vi "Controller Open Ethercat Variables.vi"(8 "error in (no error)":errorcluster, 11 "FOFB Configuration":T3={"FOFB Parameters"={"Network"={"FOFB Controller IP"="", "LNLS Control Network IP"="", "LNLS Control Network Power Supplies TCP Port"=0, "LNLS Control Network FOFB Configuration TCP Port"=0, "Data Server TCP Port"=0, "Monitoring Data TCP Port"=0, "Configuration GUI TCP Port"=0, "TCP Listening Timeout"=0}, "Fast Acquisition"={"Acquisition Period"=0, "Data Buffer Size"=0, "Monitoring Period"=0}, "Response Matrix Measurement"={"Step Amplitude"=0.0, "Time Between Steps"=0, "Step Duration"=0, "Number of Averages"=0}, "Correction Algorithm"={"Correction Period"=0, "Reference Orbit Path"=path "", "Response Matrix Path"=path "", "Correction Matrix Path"=path "", "Horizontal Correction Factor"=0.0, "Vertical Correction Factor"=0.0, "Beam Current FOFB Threshold"=0.0, "Decouple H-V"=FALSE, "Use Additional BPM LPF"=FALSE, "BPM LPF Cutoff"=0.0}, "Acquisition Network"=[], "Actuation Network"=[]}, "Number of Acquisition Chassis"=0, "Number of Actuation Chassis"=0, "Number of BPM Readings"=0, "BPM Reading Names"=[], "Selected BPM Readings"=[0, 1, 2, 3, 4, 5, 6, 7, 8, 9, 10, 11, 12, 13, 14, 15, 16, 17, 18, 19, 20, 21, 22, 23, 24, 25, 26, 27, 28, 29, 30, 31, 32, 33, 34, 35, 36, 37, 38, 39, 40, 41, 42, 43, 44, 45, 46, 47, 48, 49], "Number of Correctors"=0, "Corrector Names"=[], "Selected Correctors"=[0, 1, 2, 3, 4, 5, 6, 7, 8, 9, 10, 11, 12, 13, 14, 15, 16, 17, 18, 19, 20, 21, 22, 23, 24, 25, 26, 27, 28, 29, 30, 31, 32, 33, 34, 35, 36, 37, 38, 39, 40, 41, 42, 43, 44, 45, 46, 47, 48, 49], "Reference Orbit"=[], "Response Matrix"=[], "Correction Matrix"=[], "Acquisition Chassis Names"=[], "Actuation Chassis Names"=[], "Acquisition Variables"=[], "Actuation Variables"=[], "PS Matrix Mapping"=[], "Inverse PS Matrix Mapping"=[], "Response Matrix Beam Energy (MeV)"=0.0, "PID Parameters"=[], "BPM Planes"=[], "Corrector Planes"=[], "RMM Step Factor"=[]}) -> (0 "error out":errorcluster, 2 "PS Variables":T1, 3 "BPM Variables":T2)   [LabVIEW 2011, in "Controller VIs.lvlib"]
doc: "Open references for all Acquisition and Actuation variables which are used to exchange data between the FOFB Controller and the Acquisition/Actuation chassis via the EtherCAT networks."
uses:
  Controller VIs.lvlib
  Types Definitions/Type FOFB Configuration.ctl
  Types Definitions/Type FOFB Parameters.ctl
  Types Definitions/Type Network Configuration.ctl
  Types Definitions/Type FA Configuration.ctl
  Types Definitions/Type Response Matrix Measurement Configuration.ctl
  Types Definitions/Type Correction Algorithm Configuration.ctl
  Types Definitions/Type Acquisition Network Configuration.ctl
  Types Definitions/Type Actuation Network Configuration.ctl
  Types Definitions/Type PID Parameters.ctl
  Types Definitions/Type BPM Variables.ctl
  Types Definitions/Type PS Variables.ctl
  Type Definitions.lvlib
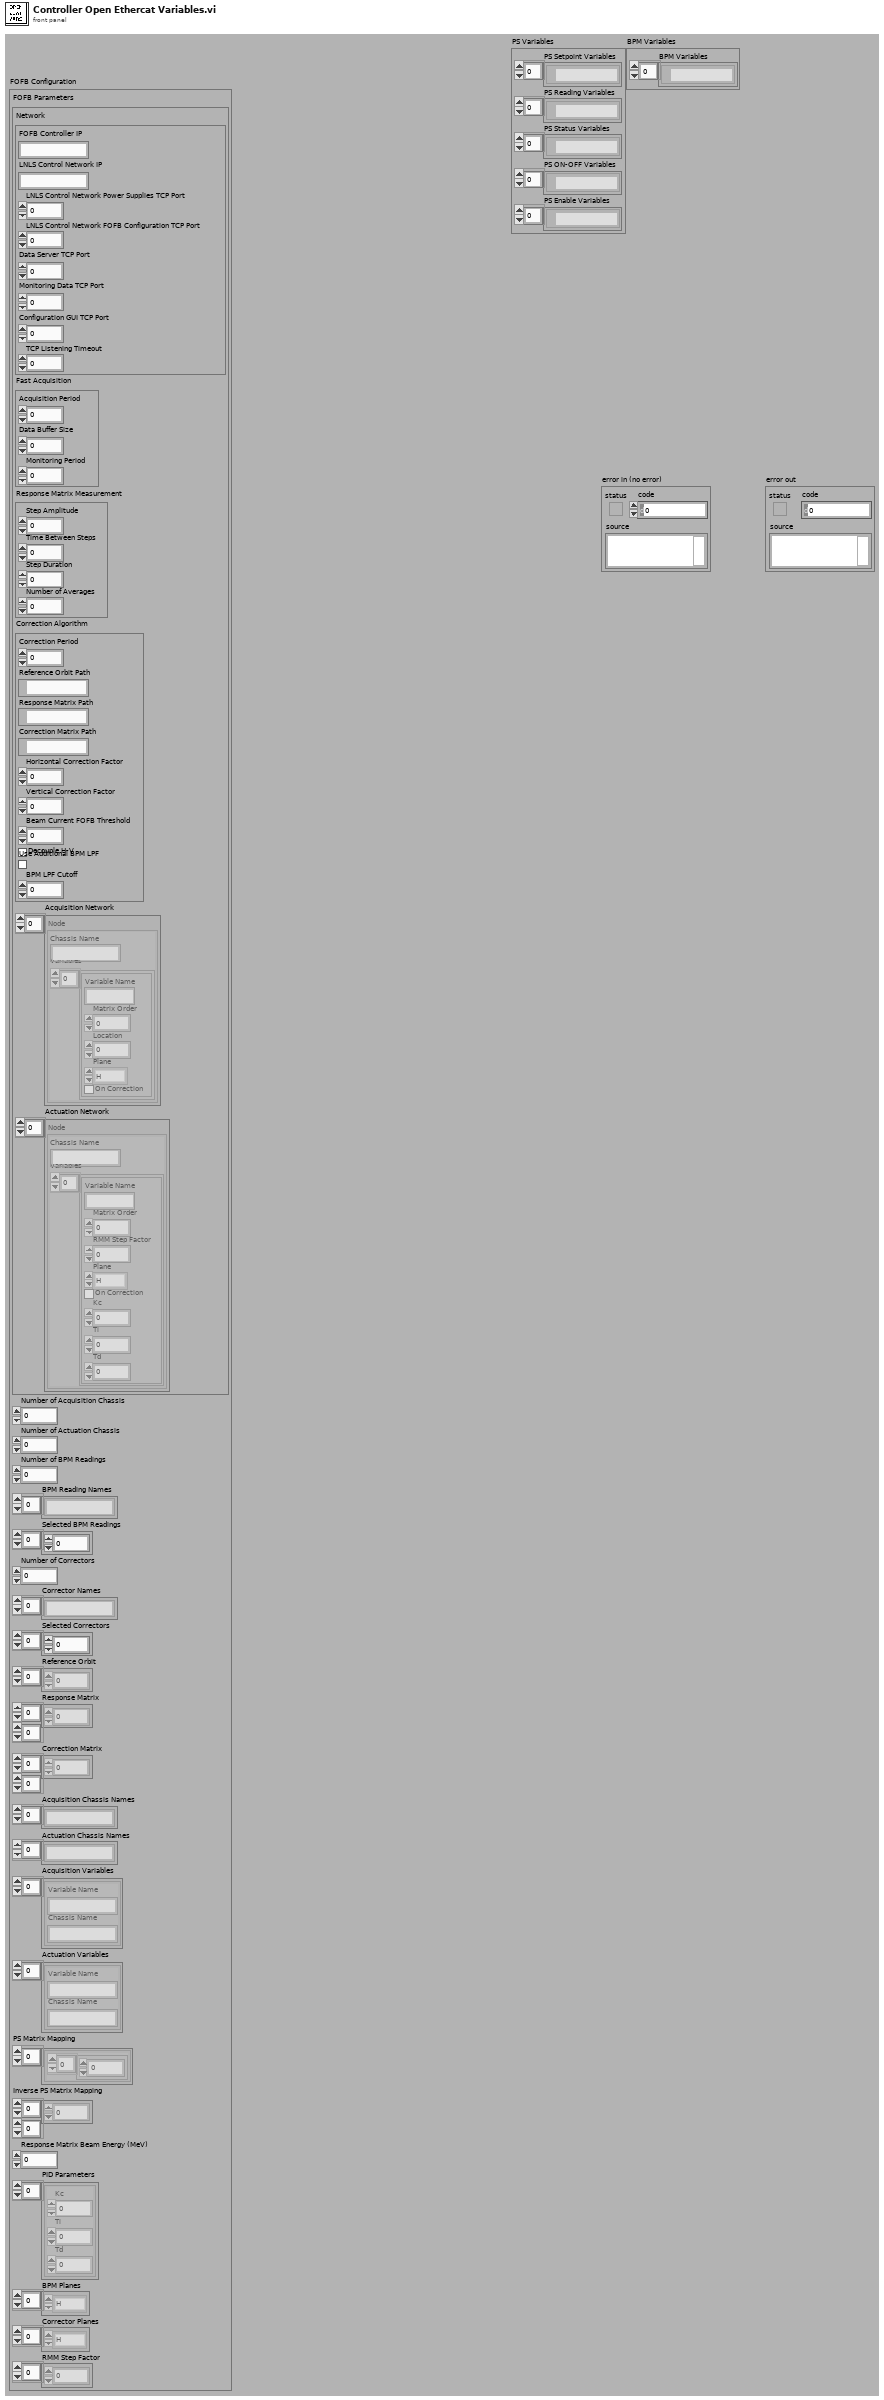
[diagram p1: front panel]
types:
  T1 = typedef "Type Definitions.lvlib/Type PS Variables.ctl" = cluster{"PS Setpoint Variables":refnum<k21>[], "PS Reading Variables":refnum<k21>[], "PS Status Variables":refnum<k21>[], "PS ON-OFF Variables":refnum<k21>[], "PS Enable Variables":refnum<k21>[]}
  T2 = typedef "Type Definitions.lvlib/Type BPM Variables.ctl" = cluster{"BPM Variables":refnum<k21>[]}
  T3 = typedef "Type Definitions.lvlib/Type FOFB Configuration.ctl" = cluster{"FOFB Parameters":T4, "Number of Acquisition Chassis":i32, "Number of Actuation Chassis":i32, "Number of BPM Readings":i32, "BPM Reading Names":string[], "Selected BPM Readings":u32[], "Number of Correctors":i32, "Corrector Names":string[], "Selected Correctors":u32[], "Reference Orbit":dbl[], "Response Matrix":dbl[][], "Correction Matrix":dbl[][], "Acquisition Chassis Names":string[], "Actuation Chassis Names":string[], "Acquisition Variables":cluster{"Variable Name":string, "Chassis Name":string}[], "Actuation Variables":cluster{"Variable Name":string, "Chassis Name":string}[], "PS Matrix Mapping":cluster{u32[]}[], "Inverse PS Matrix Mapping":u32[][], "Response Matrix Beam Energy (MeV)":dbl, "PID Parameters":T11[], "BPM Planes":enum8{"H", "V"}[], "Corrector Planes":enum8{"H", "V"}[], "RMM Step Factor":dbl[]}
  T4 = typedef "Type Definitions.lvlib/Type FOFB Parameters.ctl" = cluster{"Network":T5, "Fast Acquisition":T6, "Response Matrix Measurement":T7, "Correction Algorithm":T8, "Acquisition Network":T9, "Actuation Network":T10}
  T5 = typedef "Type Definitions.lvlib/Type Network Configuration.ctl" = cluster{"FOFB Controller IP":string, "LNLS Control Network IP":string, "LNLS Control Network Power Supplies TCP Port":u16, "LNLS Control Network FOFB Configuration TCP Port":u16, "Data Server TCP Port":u16, "Monitoring Data TCP Port":u16, "Configuration GUI TCP Port":u16, "TCP Listening Timeout":i32}
  T6 = typedef "Type Definitions.lvlib/Type FA Configuration.ctl" = cluster{"Acquisition Period":u32, "Data Buffer Size":u32, "Monitoring Period":u32}
  T7 = typedef "Type Definitions.lvlib/Type Response Matrix Measurement Configuration.ctl" = cluster{"Step Amplitude":dbl, "Time Between Steps":u32, "Step Duration":u32, "Number of Averages":u32}
  T8 = typedef "Type Definitions.lvlib/Type Correction Algorithm Configuration.ctl" = cluster{"Correction Period":u32, "Reference Orbit Path":path, "Response Matrix Path":path, "Correction Matrix Path":path, "Horizontal Correction Factor":dbl, "Vertical Correction Factor":dbl, "Beam Current FOFB Threshold":dbl, "Decouple H-V":bool, "Use Additional BPM LPF":bool, "BPM LPF Cutoff":dbl}
  T9 = typedef "Type Definitions.lvlib/Type Acquisition Network Configuration.ctl" = cluster{"Chassis Name":string, "Variables":cluster{"Variable Name":string, "Matrix Order":u32, "Location":dbl, "Plane":enum8{"H", "V"}, "On Correction":bool}[]}[]
  T10 = typedef "Type Definitions.lvlib/Type Actuation Network Configuration.ctl" = cluster{"Chassis Name":string, "Variables":cluster{"Variable Name":string, "Matrix Order":u32, "RMM Step Factor":dbl, "Plane":enum8{"H", "V"}, "On Correction":bool, "Kc":dbl, "Ti":dbl, "Td":dbl}[]}[]
  T11 = typedef "Type Definitions.lvlib/Type PID Parameters.ctl" = cluster{"Kc":fxp<+/-,16,8>, "Ti":fxp<+/-,16,8>, "Td":fxp<+/-,16,8>}
  T12 = cluster{"Variable Name":string, "Chassis Name":string}[]
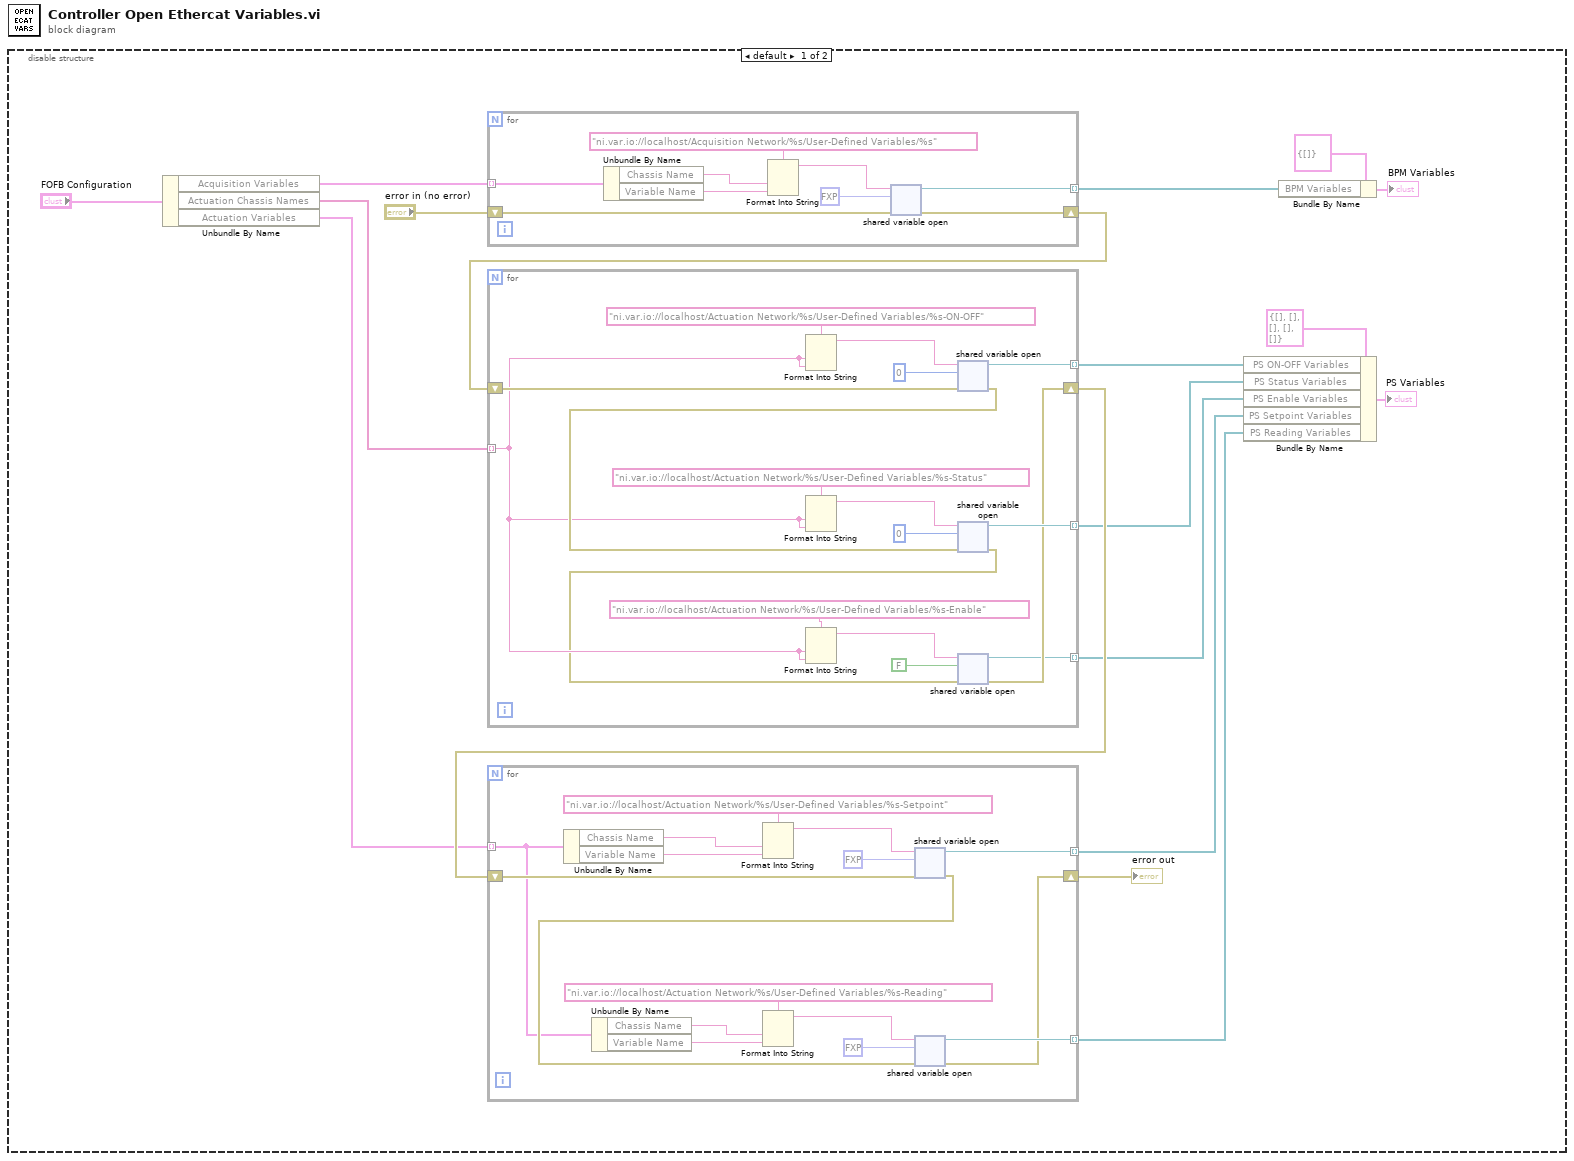
[diagram p0: block diagram]
diagram:
  n1 = disable-structure shown="default" {
    frame condition #0 {
      n2 = Unbundle By Name("FOFB Configuration") -> ("Acquisition Variables"=w8:T12, "Actuation Chassis Names"=w7:string[], "Actuation Variables"=w6:T12)
      n3 = for {
        tunnel: w8 -> [w54] mode=indexing
        shift-right: [w59] -> w13
        shift-left: "error in (no error)" -> [w58]
        tunnel: [w57] -> w17 mode=indexing
        n4 = Unbundle By Name(w54) -> ("Chassis Name"=w53:string, "Variable Name"=w52:string)
        n5 = Format Into String(format string="ni.var.io://localhost/Acquisition Network/%s/User-Defined Variables/%s", w53, w52) -> (resulting string=w56:string)  [unwired: 2 in, 1 out]
        n6 = shared-variable-open(w56, w58, fxp<+/-,20,5> 0.0 ("BPM Data")) -> (w57:refnum<k21>, w59:errorcluster)  [unwired: 1 in]
      }
      n7 = for {
        shift-right: [w20] -> w12
        shift-left: w13 -> [w28]
        tunnel: w7 -> [w22] mode=indexing
        tunnel: [w27] -> w11 mode=indexing
        tunnel: [w26] -> w10 mode=indexing
        tunnel: [w19] -> w3 mode=indexing
        n8 = Format Into String(format string="ni.var.io://localhost/Actuation Network/%s/User-Defined Variables/%s-ON-OFF", w22, w22) -> (resulting string=w35:string)  [unwired: 2 in, 1 out]
        n9 = Format Into String(format string="ni.var.io://localhost/Actuation Network/%s/User-Defined Variables/%s-Status", w22, w22) -> (resulting string=w32:string)  [unwired: 2 in, 1 out]
        n10 = Format Into String(format string="ni.var.io://localhost/Actuation Network/%s/User-Defined Variables/%s-Enable", w22, w22) -> (resulting string=w24:string)  [unwired: 2 in, 1 out]
        n11 = shared-variable-open(w35, w28, u8 0) -> (w27:refnum<k21>, w31:errorcluster)  [unwired: 1 in]
        n12 = shared-variable-open(w32, w31, u8 0) -> (w26:refnum<k21>, w21:errorcluster)  [unwired: 1 in]
        n13 = shared-variable-open(w24, w21, FALSE) -> (w19:refnum<k21>, w20:errorcluster)  [unwired: 1 in]
      }
      n14 = for {
        shift-right: [w41] -> w15
        shift-left: w12 -> [w42]
        tunnel: w6 -> [w38] mode=indexing
        tunnel: [w46] -> w4 mode=indexing
        tunnel: [w45] -> w9 mode=indexing
        n15 = Unbundle By Name(w38) -> ("Chassis Name"=w40:string, "Variable Name"=w39:string)
        n16 = Unbundle By Name(w38) -> ("Chassis Name"=w36:string, "Variable Name"=w37:string)
        n17 = Format Into String(format string="ni.var.io://localhost/Actuation Network/%s/User-Defined Variables/%s-Setpoint", w40, w39) -> (resulting string=w51:string)  [unwired: 2 in, 1 out]
        n18 = Format Into String(format string="ni.var.io://localhost/Actuation Network/%s/User-Defined Variables/%s-Reading", w36, w37) -> (resulting string=w48:string)  [unwired: 2 in, 1 out]
        n19 = shared-variable-open(w51, w42, fxp<+/-,20,5> 0.0 ("PS Setpoint Data")) -> (w46:refnum<k21>, w47:errorcluster)  [unwired: 1 in]
        n20 = shared-variable-open(w48, w47, fxp<+/-,20,5> 0.0 ("PS Reading Data")) -> (w45:refnum<k21>, w41:errorcluster)  [unwired: 1 in]
      }
      "error out" <- w15
      n21 = Bundle By Name(cluster=T1 {"PS Setpoint Variables"=[], "PS Reading Variables"=[], "PS Status Variables"=[], "PS ON-OFF Variables"=[], "PS Enable Variables"=[]} ("output cluster"), "PS ON-OFF Variables"=w11, "PS Status Variables"=w10, "PS Enable Variables"=w3, "PS Setpoint Variables"=w4, "PS Reading Variables"=w9) -> (→"PS Variables":T1)
      n22 = Bundle By Name(cluster=T2 {"BPM Variables"=[]} ("output cluster"), "BPM Variables"=w17) -> (→"BPM Variables":T2)
    }
    frame condition #1 (active) {
    }
  }
